vi "Set WinBottom.vi"(8 "error in (no error)":errorcluster, 11 "hWnd":u32) -> (0 "error out":errorcluster)   [LabVIEW 2025, in "Test Unit.lvlib"]
uses:
  Test Unit.lvlib
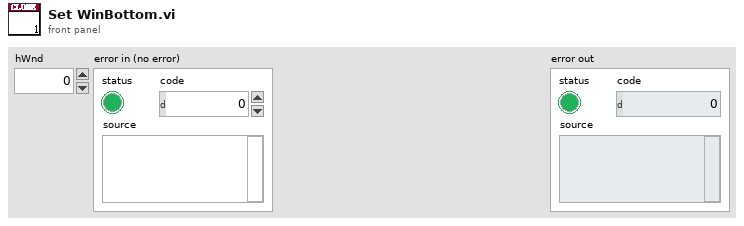
[diagram p1: front panel]
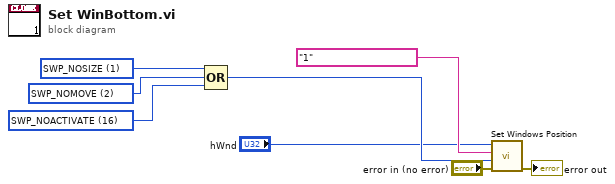
[diagram p0: block diagram]
diagram:
  w5 = u32 16 items=["SWP_ASYNCWINDOWPOS"=16384, "SWP_DEFERERASE"=8192, "SWP_DRAWFRAME"=32, "SWP_HIDEWINDOW"=128, "SWP_NOACTIVATE"=16, "SWP_NOCOPYBITS"=256, "SWP_NOMOVE"=2, "SWP_NOOWNERZORDER"=512, "SWP_NOREDRAW"=8, "SWP_NOSENDCHANGING"=1024, "SWP_NOSIZE"=1, "SWP_NOZORDER"=4, "SWP_SHOWWINDOW"=64] ("uFlags")
  w6 = u32 2 items=["SWP_ASYNCWINDOWPOS"=16384, "SWP_DEFERERASE"=8192, "SWP_DRAWFRAME"=32, "SWP_HIDEWINDOW"=128, "SWP_NOACTIVATE"=16, "SWP_NOCOPYBITS"=256, "SWP_NOMOVE"=2, "SWP_NOOWNERZORDER"=512, "SWP_NOREDRAW"=8, "SWP_NOSENDCHANGING"=1024, "SWP_NOSIZE"=1, "SWP_NOZORDER"=4, "SWP_SHOWWINDOW"=64] ("uFlags")
  w7 = u32 1 items=["SWP_ASYNCWINDOWPOS"=16384, "SWP_DEFERERASE"=8192, "SWP_DRAWFRAME"=32, "SWP_HIDEWINDOW"=128, "SWP_NOACTIVATE"=16, "SWP_NOCOPYBITS"=256, "SWP_NOMOVE"=2, "SWP_NOOWNERZORDER"=512, "SWP_NOREDRAW"=8, "SWP_NOSENDCHANGING"=1024, "SWP_NOSIZE"=1, "SWP_NOZORDER"=4, "SWP_SHOWWINDOW"=64] ("uFlags")
  n1 = Compound Arithmetic op=OR(w7, w6, w5) -> (w4:u32)
  n2 = call "Set Windows Position.vi"("error in (no error)"="error in (no error)", "uFlags"=w4, "hWndInsertAfter"="1", "hWnd"="hWnd") -> ("error out"=→"error out":errorcluster)  [unwired: 6 in, 1 out]
